vi "PH_Sequencer.evt call SetPPVoltage.vi"(0 "i ref in":refnum<vi>, 1 "Sequencer Inst":string="N/A", 2 "Power Unit":T1, 3 "PP Voltage [V]":dbl, 5 "error in (no error)":errorcluster) -> (14 "i ref out":refnum<vi>, 19 "error out":errorcluster)   [LabVIEW 2014, in "PH_Sequencer.lvlib"]
doc: "This VI calls the \"SetPPVoltage\" case by a simple call."
uses:
  PH_Sequencer.lvlib
  PH_Basics/PH_PP_Common/PH_PP_Common.PUs.ctl
  CS_Core/CSSystem/CoreLib/CoreLib.double 2 byte array.vi
  CS_Core/CSSystem/CoreLib/CoreLib.short 2 byte array.vi
  CS_Core/CSSystem/CoreLib/CoreLib.lvlib
  CS_Core/BaseProcess/BaseProcess.lvlib
  PH_Basics/PH_PP_Common/PH_PP_Common.lvlib
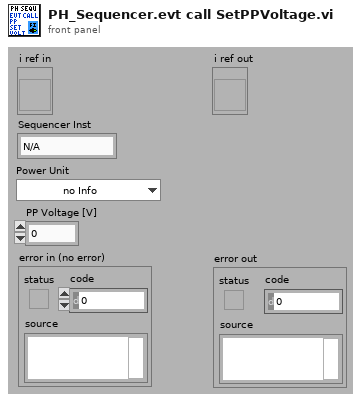
[diagram p1: front panel]
types:
  T1 = typedef "PH_PP_Common.lvlib/PH_PP_Common.PUs.ctl" = enum16{"no Info", "PA-19mm-1", "PA-19mm-2", "PA-45mm-PILC", "PA-45mm-MAIN", "MA-PU-1", "MA-PU-2", "MA-PU-3", "MA-PU-4", "MA-PU-5", "MA-PU-6", "MA-FR", "MA-PILC", "PA-45mm-DP"}
  T2 = typedef "CoreDefs.rawDataType.ctl" = i8[]
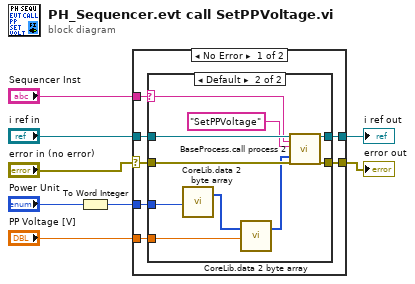
[diagram p0: block diagram]
diagram:
  n1 = To Word Integer(number="Power Unit") -> (16bit integer=w1:i16)
  n2 = case shown="No Error" "error in (no error)" {
    selector: "error in (no error)" -> [w11 w28]
    tunnel: [w15 w29] -> w3
    tunnel: [w14 w28] -> w2
    tunnel: "i ref in" -> [w13 w29]
    tunnel: "Sequencer Inst" -> [w12 _]
    tunnel: "PP Voltage [V]" -> [w10 _]
    tunnel: w1 -> [w9 _]
    frame No Error {
      n3 = case shown="Default" w12 {
        selector: w12 -> [_ w21]
        tunnel: [w17 w27] -> w15
        tunnel: [w16 w26] -> w14
        tunnel: w13 -> [w17 w25]
        tunnel: w11 -> [w16 w24]
        tunnel: w10 -> [_ w20]
        tunnel: w9 -> [_ w18]
        frame "N/A" {
        }
        frame Default {
          n4 = call-poly "CoreLib.data 2 byte array.vi"("i16"=w18) -> ("byteArray out"=w19:T2)  [unwired: 18 in]
          n5 = call-poly "CoreLib.data 2 byte array.vi"("byteArray"=w19, "f64"=w20) -> ("byteArray out"=w22:T2)  [unwired: 17 in]
          n6 = call "BaseProcess.call process 2.vi"("i ref in"=w25, "Object"=w21, "Selector"="SetPPVoltage", "Data"=w22, "error in (no error)"=w24) -> ("i ref out"=w27:refnum<vi>, "error out"=w26:errorcluster)  [unwired: 13 in]
        }
      }
    }
    frame Error {
    }
  }
  "i ref out" <- w3
  "error out" <- w2
